vi "Addition.vi"() -> ()   [LabVIEW 2018]
panel:
  out "output":dbl
  in  "2nd number":dbl
  in  "1st number":dbl
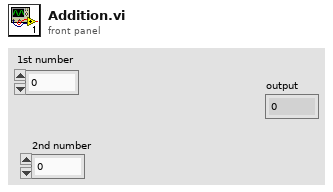
[diagram p1: front panel]
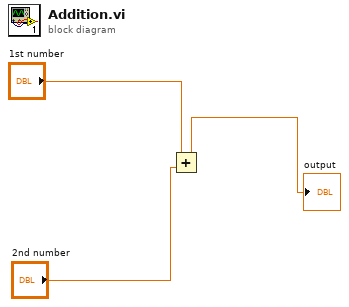
[diagram p0: block diagram]
diagram:
  n1 = Add(x="1st number", y="2nd number") -> (x+y=→"output":dbl)
